vi "Q-Switch_Delay.vi"(8 "error in (no error)":errorcluster, 10 "Delay (us)":i32, 11 "VISA resource name":refnum<visa-resource-name>) -> (0 "error out":errorcluster, 3 "VISA resource name out":refnum<visa-resource-name>)   [LabVIEW 2012, in "Surelite I.lvlib"]
doc: "Resets the instrument and then sends a set of default setup commands to the instrument."
uses:
  Surelite I.lvlib
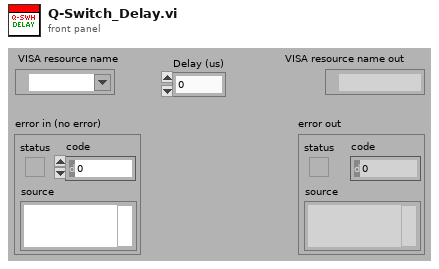
[diagram p1: front panel]
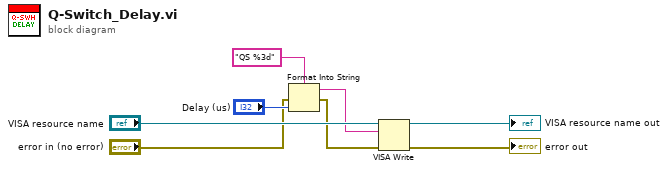
[diagram p0: block diagram]
diagram:
  n1 = Format Into String(format string="QS %3d", error in="error in (no error)", "Delay (us)") -> (resulting string=w1:string, error out=w2:errorcluster)  [unwired: 1 in]
  n2 = VISA Write(VISA resource name="VISA resource name", write buffer=w1, error in (no error)=w2) -> (VISA resource name out=→"VISA resource name out":refnum<visa-resource-name>, error out=→"error out":errorcluster)  [unwired: 1 out]
